vi "Coefficients-2.vi"() -> (0 "filter coefficients":dbl[](array[numeric]) format="%.2f")   [LabVIEW 2023]
uses:
  <vilib>/Analysis/NI_AALBase.lvlib
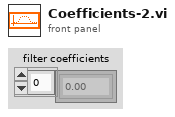
[diagram p1: front panel]
types:
  T1 = cluster{"Amplitude":dbl, "Lower Freq":dbl, "Higher Freq":dbl, "Weighted\nRipple":dbl}[]
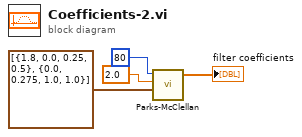
[diagram p0: block diagram]
diagram:
  n1 = call <vilib>:"Parks-McClellan.vi"("Band Parameters"=T1 [{"Amplitude"=1.8, "Lower Freq"=0.0, "Higher Freq"=0.25, "Weighted\nRipple"=0.5}, {"Amplitude"=0.0, "Lower Freq"=0.275, "Higher Freq"=1.0, "Weighted\nRipple"=1.0}], "sampling freq: fs"=2.0, "# of taps"=80) -> ("h"=→"filter coefficients":dbl[])  [unwired: 1 in, 2 out]
